vi "rszvl_core_global.vi"() -> ()   [LabVIEW 2014] (continued)
L8\r\nModifMinMaxAver: Min,Max,Aver\r\n\nRemote-control command(s):\nCALCulate<1|2>:LIMit<1>:BURSt:EVM:DATA<[:AVERage] | :MAXimum>", "Flags"={"OPC Wait"=FALSE, "Dont check status"=FALSE, "*WAI"=FALSE}, "Check Status Callback"=""}, {"Level"=3, "Descriptive Name"="WLAN Pilot Carrier EVM Limit", "Class Only"=FALSE, "Data Type"=1, "Access"=2, "Identifier"="RSZVL_ATTR_WLAN_EVM_PIL", "Range Table"="", "Command"="CALC{Window}:LIM{Limit}:BURS:EVM:PIL:{ModifMinMaxAver}", "Read Callback"="", "Write Callback"="", "Range Callback"="", "Check Callback"="", "Rngtable Callback"="", "Coerce Callback"="", "User Callback"="", "Supported Models"="", "Instrument Options"="", "Repeated Capabilities"="", "Restricted Repeated Capabilities"="", "Help"="This attribute sets the Error Vector Magnitude limit summary for the pilot carriers in dB.\n\nAvailable Repeated Capabilities:\nWindow: Win1,Win2\r\nLimit: L1,L2,L3,L4,L5,L6,L7,L8\r\nModifMinMaxAver: Min,Max,Aver\r\n\nRemote-control command(s):\nCALCulate<1|2>:LIMit<1>:BURSt:EVM:PILot<[:AVERage] | :MAXimum>", "Flags"={"OPC Wait"=FALSE, "Dont check status"=FALSE, "*WAI"=FALSE}, "Check Status Callback"=""}, {"Level"=2, "Descriptive Name"="Limit Results", "Class Only"=TRUE, "Data Type"=0, "Access"=0, "Identifier"="", "Range Table"="", "Command"="", "Read Callback"="", "Write Callback"="", "Range Callback"="", "Check Callback"="", "Rngtable Callback"="", "Coerce Callback"="", "User Callback"="", "Supported Models"="", "Instrument Options"="", "Repeated Capabilities"="", "Restricted Repeated Capabilities"="", "Help"="Attributes that return the limit results.\n\n(1) WLAN Get Fall Time Limit Result:\nThis attribute returns the fall time limit result.\n\nNote:\n(1) This attribute is valid only if standard IEEE 802.11b is selected.\n\n(2) WLAN Get Rise Time Limit Result:\nThis attribute returns the rise time limit result.\n\nNote:\n(1) This attribute is valid only if standard IEEE 802.11b is selected.\n\n(3) WLAN Get Frequency Error Limit Result:\nThis attribute returns the frequency error limit result.\n\n(4) WLAN Get Symbol Error Limit Result:\nThis attribute returns the symbol error limit result.\n\n(5) WLAN Get IQ Offset Error Limit Result:\nThis attribute returns the IQ offset error limit result.\n\n(6) WLAN Get Error Vector Magnitude Limit Result:\nThis attribute returns the Error Vector Magnitude Limit result.\n\nNote:\n(1) This attribute is available only for IEEE 802.11b standard.\n\n(7) WLAN Get Limit Check Result:\nThis attribute queries the result of the limit check of the limit line indicated in the selected\nmeasurement window. The result of the limit check responds with 0 for PASS and 1 for FAIL.\n\n\n\n(8) WLAN Get Combined EVM Limit Result:\nThis attribute returns the Error Vector Magnitude Limit result. This is a combined figure that represents the pilot, data and the free carrier.\n\n(9) WLAN Get Data Carrier EVM Limit Result:\nThis attribute returns the Error Vector Magnitude limit result summary for the data carrier in dB.\n\nValid Range:\n0 - Failed\n1 - Passed\n\n(10) WLAN Get Pilot Carrier EVM Limit Result:\nThis attribute returns the Error Vector Magnitude limit result summary for the pilot carriers in dB.\n\nValid Range:\n0 - Failed\n1 - Passed\n\n(11) WLAN Get ACP Adjacent Channel Limit:\nThis attribute returns the ACP adjacent channel limit.\n\nNote:\n(1) This attribute is available only if IEEE 802.11j is defined.\n\n(12) WLAN Get ACP Adjacent Channel Limit Result:\nThis attribute returns the ACP adjacent channel limit for IEEE 802.11j result summary (PASSED |\nFAILED) for both the lower and upper adjacent channels.\n\nNote:\n(1) This attribute is available only if IEEE 802.11j is defined.\n\n(13) WLAN Get ACP Alternate Channel Limit:\nThis attribute returns the ACP alternate channel limit.\n\nNote:\n(1) This attribute is available only if IEEE 802.11j is defined.\n\n(14) WLAN Get ACP Alternate Channel Limit Result:\nThis attribute returns the returns the ACP alternate channel limit result.\n\nNote:\n(1) This attribute is available only if IEEE 802.11j is defined.\n\n(15) WLAN Get Spectrum Max Oversteping Frequency:\nThis attribute returns the X-value at the maximum overstepping of the spectrum mask limits.\n\n(16) WLAN Get Spectrum Max Oversteping Power:\nThis attribute returns the Y-value at the maximum overstepping of the spectrum mask limits.", "Flags"={"OPC Wait"=FALSE, "Dont check status"=FALSE, "*WAI"=FALSE}, "Check Status Callback"=""}, {"Level"=3, "Descriptive Name"="WLAN Get Fall Time Limit Result", "Class Only"=FALSE, "Data Type"=0, "Access"=0, "Identifier"="RSZVL_ATTR_WLAN_TFAL_RES", "Range Table"="rszvl_rngResults", "Command"="CALC{Window}:LIM{Limit}:BURS:TFALl:{ModifMinMaxAver}:RES?", "Read Callback"="", "Write Callback"="", "Range Callback"="", "Check Callback"="", "Rngtable Callback"="", "Coerce Callback"="", "User Callback"="", "Supported Models"="", "Instrument Options"="", "Repeated Capabilities"="", "Restricted Repeated Capabilities"="", "Help"="This attribute returns the fall time limit result.\n\nNote:\n(1) This attribute is valid only if standard IEEE 802.11b is selected.\n\nAvailable Repeated Capabilities:\nWindow: Win1,Win2\r\nLimit: L1,L2,L3,L4,L5,L6,L7,L8\r\nModifMinMaxAver: Min,Max,Aver\r\n\nRemote-control command(s):\nCALCulate<1|2>:LIMit<1>:BURSt:TFALl<[:AVERage] | :MAXimum>:RESult?", "Flags"={"OPC Wait"=FALSE, "Dont check status"=FALSE, "*WAI"=FALSE}, "Check Status Callback"=""}, {"Level"=3, "Descriptive Name"="WLAN Get Rise Time Limit Result", "Class Only"=FALSE, "Data Type"=0, "Access"=0, "Identifier"="RSZVL_ATTR_WLAN_TRIS_RES", "Range Table"="rszvl_rngResults", "Command"="CALC{Window}:LIM{Limit}:BURS:TRIS:{ModifMinMaxAver}:RES?", "Read Callback"="", "Write Callback"="", "Range Callback"="", "Check Callback"="", "Rngtable Callback"="", "Coerce Callback"="", "User Callback"="", "Supported Models"="", "Instrument Options"="", "Repeated Capabilities"="", "Restricted Repeated Capabilities"="", "Help"="This attribute returns the rise time limit result.\n\nNote:\n(1) This attribute is valid only if standard IEEE 802.11b is selected.\n\nAvailable Repeated Capabilities:\nWindow: Win1,Win2\r\nLimit: L1,L2,L3,L4,L5,L6,L7,L8\r\nModifMinMaxAver: Min,Max,Aver\r\n\nRemote-control command(s):\nCALCulate<1|2>:LIMit<1>:BURSt:TRISe<[:AVERage] | :MAXimum>:RESult?", "Flags"={"OPC Wait"=FALSE, "Dont check status"=FALSE, "*WAI"=FALSE}, "Check Status Callback"=""}, {"Level"=3, "Descriptive Name"="WLAN Get Frequency Error Limit Result", "Class Only"=FALSE, "Data Type"=0, "Access"=0, "Identifier"="RSZVL_ATTR_WLAN_FERR_RES", "Range Table"="rszvl_rngResults", "Command"="CALC{Window}:LIM{Limit}:BURS:FERR:{ModifMinMaxAver}:RES?", "Read Callback"="", "Write Callback"="", "Range Callback"="", "Check Callback"="", "Rngtable Callback"="", "Coerce Callback"="", "User Callback"="", "Supported Models"="", "Instrument Options"="", "Repeated Capabilities"="", "Restricted Repeated Capabilities"="", "Help"="This attribute returns the frequency error limit result.\n\nAvailable Repeated Capabilities:\nWindow: Win1,Win2\r\nLimit: L1,L2,L3,L4,L5,L6,L7,L8\r\nModifMinMaxAver: Min,Max,Aver\r\n\nRemote-control command(s):\nCALCulate<1|2>:LIMit<1>:BURSt:FERRor<[:AVERage] | :MAXimum>:RESult?", "Flags"={"OPC Wait"=FALSE, "Dont check status"=FALSE, "*WAI"=FALSE}, "Check Status Callback"=""}, {"Level"=3, "Descriptive Name"="WLAN Get Symbol Error Limit Result", "Class Only"=FALSE, "Data Type"=0, "Access"=0, "Identifier"="RSZVL_ATTR_WLAN_SYMB_RES", "Range Table"="rszvl_rngResults", "Command"="CALC{Window}:LIM{Limit}:BURS:SYMB:{ModifMinMaxAver}:RES?", "Read Callback"="", "Write Callback"="", "Range Callback"="", "Check Callback"="", "Rngtable Callback"="", "Coerce Callback"="", "User Callback"="", "Supported Models"="", "Instrument Options"="", "Repeated Capabilities"="", "Restricted Repeated Capabilities"="", "Help"="This attribute returns the symbol error limit result.\n\nAvailable Repeated Capabilities:\nWindow: Win1,Win2\r\nLimit: L1,L2,L3,L4,L5,L6,L7,L8\r\nModifMinMaxAver: Min,Max,Aver\r\n\nRemote-control command(s):\nCALCulate<1|2>:LIMit<1>:BURSt:SYMBolerror<[:AVERage] | :MAXimum>:RESult?", "Flags"={"OPC Wait"=FALSE, "Dont check status"=FALSE, "*WAI"=FALSE}, "Check Status Callback"=""}, {"Level"=3, "Descriptive Name"="WLAN Get IQ Offset Error Limit Result", "Class Only"=FALSE, "Data Type"=0, "Access"=0, "Identifier"="RSZVL_ATTR_WLAN_IQOF_RES", "Range Table"="rszvl_rngResults", "Command"="CALC{Window}:LIM{Limit}:BURS:IQOF:{ModifMinMaxAver}:RES?", "Read Callback"="", "Write Callback"="", "Range Callback"="", "Check Callback"="", "Rngtable Callback"="", "Coerce Callback"="", "User Callback"="", "Supported Models"="", "Instrument Options"="", "Repeated Capabilities"="", "Restricted Repeated Capabilities"="", "Help"="This attribute returns the IQ offset error limit result.\n\nAvailable Repeated Capabilities:\nWindow: Win1,Win2\r\nLimit: L1,L2,L3,L4,L5,L6,L7,L8\r\nModifMinMaxAver: Min,Max,Aver\r\n\nRemote-control command(s):\nCALCulate<1|2>:LIMit<1>:BURSt:IQOFfset<[:AVERage] | :MAXimum>:RESult?", "Flags"={"OPC Wait"=FALSE, "Dont check status"=FALSE, "*WAI"=FALSE}, "Check Status Callback"=""}, {"Level"=3, "Descriptive Name"="WLAN Get Error Vector Magnitude Limit Result", "Class Only"=FALSE, "Data Type"=0, "Access"=0, "Identifier"="RSZVL_ATTR_WLAN_EVM_RES", "Range Table"="rszvl_rngResults", "Command"="CALC{Window}:LIM{Limit}:BURS:EVM:{ModifMinMaxAver}:RES?", "Read Callback"="", "Write Callback"="", "Range Callback"="", "Check Callback"="", "Rngtable Callback"="", "Coerce Callback"="", "User Callback"="", "Supported Models"="", "Instrument Options"="", "Repeated Capabilities"="", "Restricted Repeated Capabilities"="", "Help"="This attribute returns the Error Vector Magnitude Limit result.\n\nNote:\n(1) This attribute is available only for IEEE 802.11b standard.\n\nAvailable Repeated Capabilities:\nWindow: Win1,Win2\r\nLimit: L1,L2,L3,L4,L5,L6,L7,L8\r\nModifMinMaxAver: Min,Max,Aver\r\n\nRemote-control command(s):\nCALCulate<1|2>:LIMit<1>:BURSt:EVM<[:AVERage] | :MAXimum>:RESult?", "Flags"={"OPC Wait"=FALSE, "Dont check status"=FALSE, "*WAI"=FALSE}, "Check Status Callback"=""}, {"Level"=3, "Descriptive Name"="WLAN Get Limit Check Result", "Class Only"=FALSE, "Data Type"=0, "Access"=0, "Identifier"="RSZVL_ATTR_WLAN_LIM_FAIL_RES", "Range Table"="", "Command"="CALC{Window}:LIM{Limit}:FAIL?", "Read Callback"="", "Write Callback"="", "Range Callback"="", "Check Callback"="", "Rngtable Callback"="", "Coerce Callback"="", "User Callback"="", "Supported Models"="", "Instrument Options"="", "Repeated Capabilities"="", "Restricted Repeated Capabilities"="", "Help"="This attribute queries the result of the limit check of the limit line indicated in the selected\nmeasurement window. The result of the limit check responds with 0 for PASS and 1 for FAIL.\n\nAvailable Repeated Capabilities:\nWindow: Win1,Win2\r\nLimit: L1,L2,L3,L4,L5,L6,L7,L8\r\n\nRemote-control command(s):\nCALCulate<1|2>:LIMit<1>:FAIL?", "Flags"={"OPC Wait"=FALSE, "Dont check status"=FALSE, "*WAI"=FALSE}, "Check Status Callback"=""}, {"Level"=3, "Descriptive Name"="WLAN Get Combined EVM Limit Result", "Class Only"=FALSE, "Data Type"=0, "Access"=0, "Identifier"="RSZVL_ATTR_WLAN_EVM_ALL_RES", "Range Table"="rszvl_rngResults", "Command"="CALC{Window}:LIM{Limit}:BURS:EVM:ALL:{ModifMinMaxAver}:RES?", "Read Callback"="", "Write Callback"="", "Range Callback"="", "Check Callback"="", "Rngtable Callback"="", "Coerce Callback"="", "User Callback"="", "Supported Models"="", "Instrument Options"="", "Repeated Capabilities"="", "Restricted Repeated Capabilities"="", "Help"="This attribute returns the Error Vector Magnitude Limit result. This is a combined figure that represents the pilot, data and the free carrier.\n\nAvailable Repeated Capabilities:\nWindow: Win1,Win2\r\nLimit: L1,L2,L3,L4,L5,L6,L7,L8\r\nModifMinMaxAver: Min,Max,Aver\r\n\nRemote-control command(s):\nCALCulate<1|2>:LIMit<1>:BURSt:EVM:ALL<[:AVERage] | :MAXimum>:RESult?", "Flags"={"OPC Wait"=FALSE, "Dont check status"=FALSE, "*WAI"=FALSE}, "Check Status Callback"=""}, {"Level"=3, "Descriptive Name"="WLAN Get Data Carrier EVM Limit Result", "Class Only"=FALSE, "Data Type"=0, "Access"=0, "Identifier"="RSZVL_ATTR_WLAN_EVM_DATA_RES", "Range Table"="rszvl_rngResults", "Command"="CALC{Window}:LIM{Limit}:BURS:EVM:DATA:{ModifMinMaxAver}:RES?", "Read Callback"="", "Write Callback"="", "Range Callback"="", "Check Callback"="", "Rngtable Callback"="", "Coerce Callback"="", "User Callback"="", "Supported Models"="", "Instrument Options"="", "Repeated Capabilities"="", "Restricted Repeated Capabilities"="", "Help"="This attribute returns the Error Vector Magnitude limit result summary for the data carrier in dB.\n\nValid Range:\n0 - Failed\n1 - Passed\n\nAvailable Repeated Capabilities:\nWindow: Win1,Win2\r\nLimit: L1,L2,L3,L4,L5,L6,L7,L8\r\nModifMinMaxAver: Min,Max,Aver\r\n\nRemote-control command(s):\nCALCulate<1|2>:LIMit<1>:BURSt:EVM:DATA<[:AVERage] | :MAXimum>:RESult?", "Flags"={"OPC Wait"=FALSE, "Dont check status"=FALSE, "*WAI"=FALSE}, "Check Status Callback"=""}, {"Level"=3, "Descriptive Name"="WLAN Get Pilot Carrier EVM Limit Result", "Class Only"=FALSE, "Data Type"=0, "Access"=0, "Identifier"="RSZVL_ATTR_WLAN_EVM_PIL_RES", "Range Table"="rszvl_rngResults", "Command"="CALC{Window}:LIM{Limit}:BURS:EVM:PIL:{ModifMinMaxAver}:RES?", "Read Callback"="", "Write Callback"="", "Range Callback"="", "Check Callback"="", "Rngtable Callback"="", "Coerce Callback"="", "User Callback"="", "Supported Models"="", "Instrument Options"="", "Repeated Capabilities"="", "Restricted Repeated Capabilities"="", "Help"="This attribute returns the Error Vector Magnitude limit result summary for the pilot carriers in dB.\n\nValid Range:\n0 - Failed\n1 - Passed\n\nAvailable Repeated Capabilities:\nWindow: Win1,Win2\r\nLimit: L1,L2,L3,L4,L5,L6,L7,L8\r\nModifMinMaxAver: Min,Max,Aver\r\n\nRemote-control command(s):\nCALCulate<1|2>:LIMit<1>:BURSt:EVM:PILot<[:AVERage] | :MAXimum>:RESult?", "Flags"={"OPC Wait"=FALSE, "Dont check status"=FALSE, "*WAI"=FALSE}, "Check Status Callback"=""}, {"Level"=3, "Descriptive Name"="WLAN Get ACP Adjacent Channel Limit", "Class Only"=FALSE, "Data Type"=1, "Access"=0, "Identifier"="RSZVL_ATTR_WLAN_ACP_ADJ", "Range Table"="", "Command"="CALC{Window}:LIM{Limit}:ACP:ACH?", "Read Callback"="", "Write Callback"="", "Range Callback"="", "Check Callback"="", "Rngtable Callback"="", "Coerce Callback"="", "User Callback"="", "Supported Models"="", "Instrument Options"="", "Repeated Capabilities"="", "Restricted Repeated Capabilities"="", "Help"="This attribute returns the ACP adjacent channel limit.\n\nNote:\n(1) This attribute is available only if IEEE 802.11j is defined.\n\nAvailable Repeated Capabilities:\nWindow: Win1,Win2\r\nLimit: L1,L2,L3,L4,L5,L6,L7,L8\r\n\nRemote-control command(s):\nCALCulate<1|2>:LIMit<1>:ACPower:ACHannel?", "Flags"={"OPC Wait"=FALSE, "Dont check status"=FALSE, "*WAI"=FALSE}, "Check Status Callback"=""}, {"Level"=3, "Descriptive Name"="WLAN Get ACP Adjacent Channel Limit Result", "Class Only"=FALSE, "Data Type"=0, "Access"=0, "Identifier"="RSZVL_ATTR_WLAN_ACP_ADJ_RES", "Range Table"="rszvl_rngResults", "Command"="CALC{Window}:LIM{Limit}:ACP:ACH:RES?", "Read Callback"="", "Write Callback"="", "Range Callback"="", "Check Callback"="", "Rngtable Callback"="", "Coerce Callback"="", "User Callback"="", "Supported Models"="", "Instrument Options"="", "Repeated Capabilities"="", "Restricted Repeated Capabilities"="", "Help"="This attribute returns the ACP adjacent channel limit for IEEE 802.11j result summary (PASSED |\nFAILED) for both the lower and upper adjacent channels.\n\nNote:\n(1) This attribute is available only if IEEE 802.11j is defined.\n\nAvailable Repeated Capabilities:\nWindow: Win1,Win2\r\nLimit: L1,L2,L3,L4,L5,L6,L7,L8\r\n\nRemote-control command(s):\nCALCulate<1|2>:LIMit<1>:ACPower:ACHannel:RESult?", "Flags"={"OPC Wait"=FALSE, "Dont check status"=FALSE, "*WAI"=FALSE}, "Check Status Callback"=""}, {"Level"=3, "Descriptive Name"="WLAN Get ACP Alternate Channel Limit", "Class Only"=FALSE, "Data Type"=1, "Access"=0, "Identifier"="RSZVL_ATTR_WLAN_ACP_ALT", "Range Table"="", "Command"="CALC{Window}:LIM{Limit}:ACP:ALT?", "Read Callback"="", "Write Callback"="", "Range Callback"="", "Check Callback"="", "Rngtable Callback"="", "Coerce Callback"="", "User Callback"="", "Supported Models"="", "Instrument Options"="", "Repeated Capabilities"="", "Restricted Repeated Capabilities"="", "Help"="This attribute returns the ACP alternate channel limit.\n\nNote:\n(1) This attribute is available only if IEEE 802.11j is defined.\n\nAvailable Repeated Capabilities:\nWindow: Win1,Win2\r\nLimit: L1,L2,L3,L4,L5,L6,L7,L8\r\n\nRemote-control command(s):\nCALCulate<1|2>:LIMit<1>:ACPower:ALTernate?", "Flags"={"OPC Wait"=FALSE, "Dont check status"=FALSE, "*WAI"=FALSE}, "Check Status Callback"=""}, {"Level"=3, "Descriptive Name"="WLAN Get ACP Alternate Channel Limit Result", "Class Only"=FALSE, "Data Type"=0, "Access"=0, "Identifier"="RSZVL_ATTR_WLAN_ACP_ALT_RES", "Range Table"="rszvl_rngResults", "Command"="CALC{Window}:LIM{Limit}:ACP:ALT:RES?", "Read Callback"="", "Write Callback"="", "Range Callback"="", "Check Callback"="", "Rngtable Callback"="", "Coerce Callback"="", "User Callback"="", "Supported Models"="", "Instrument Options"="", "Repeated Capabilities"="", "Restricted Repeated Capabilities"="", "Help"="This attribute returns the returns the ACP alternate channel limit result.\n\nNote:\n(1) This attribute is available only if IEEE 802.11j is defined.\n\nAvailable Repeated Capabilities:\nWindow: Win1,Win2\r\nLimit: L1,L2,L3,L4,L5,L6,L7,L8\r\n\nRemote-control command(s):\nCALCulate<1|2>:LIMit<1>:ACPower:ALTernate:RESult?", "Flags"={"OPC Wait"=FALSE, "Dont check status"=FALSE, "*WAI"=FALSE}, "Check Status Callback"=""}, {"Level"=3, "Descriptive Name"="WLAN Get Spectrum Max Oversteping Frequency", "Class Only"=FALSE, "Data Type"=1, "Access"=0, "Identifier"="RSZVL_ATTR_WLAN_SPEC_MASK_X", "Range Table"="", "Command"="CALC{Window}:LIM{Limit}:SPEC:MASK:CHEC:X?", "Read Callback"="", "Write Callback"="", "Range Callback"="", "Check Callback"="", "Rngtable Callback"="", "Coerce Callback"="", "User Callback"="", "Supported Models"="", "Instrument Options"="", "Repeated Capabilities"="", "Restricted Repeated Capabilities"="", "Help"="This attribute returns the X-value at the maximum overstepping of the spectrum mask limits.\n\nAvailable Repeated Capabilities:\nWindow: Win1,Win2\r\nLimit: L1,L2,L3,L4,L5,L6,L7,L8\r\n\nRemote-control command(s):\nCALCulate<1|2>:LIMit<1>:SPECtrum:MASK:CHECk:X?", "Flags"={"OPC Wait"=FALSE, "Dont check status"=FALSE, "*WAI"=FALSE}, "Check Status Callback"=""}, {"Level"=3, "Descriptive Name"="WLAN Get Spectrum Max Oversteping Power", "Class Only"=FALSE, "Data Type"=1, "Access"=0, "Identifier"="RSZVL_ATTR_WLAN_SPEC_MASK_Y", "Range Table"="", "Command"="CALC{Window}:LIM{Limit}:SPEC:MASK:CHEC:Y?", "Read Callback"="", "Write Callback"="", "Range Callback"="", "Check Callback"="", "Rngtable Callback"="", "Coerce Callback"="", "User Callback"="", "Supported Models"="", "Instrument Options"="", "Repeated Capabilities"="", "Restricted Repeated Capabilities"="", "Help"="This attribute returns the Y-value at the maximum overstepping of the spectrum mask limits.\n\nAvailable Repeated Capabilities:\nWindow: Win1,Win2\r\nLimit: L1,L2,L3,L4,L5,L6,L7,L8\r\n\nRemote-control command(s):\nCALCulate<1|2>:LIMit<1>:SPECtrum:MASK:CHECk:Y?", "Flags"={"OPC Wait"=FALSE, "Dont check status"=FALSE, "*WAI"=FALSE}, "Check Status Callback"=""}, {"Level"=2, "Descriptive Name"="Marker Settings", "Class Only"=TRUE, "Data Type"=0, "Access"=0, "Identifier"="", "Range Table"="", "Command"="", "Read Callback"="", "Write Callback"="", "Range Callback"="", "Check Callback"="", "Rngtable Callback"="", "Coerce Callback"="", "User Callback"="", "Supported Models"="", "Instrument Options"="", "Repeated Capabilities"="", "Restricted Repeated Capabilities"="", "Help"="Attributes that configure the marker settings.\n\n(1) WLAN Marker Symbol:\nThis attribute positions the selected marker to the indicated quadrature (constellation Vs symbol), magnitude of I or Q (constellation Vs carrier), EVM (EVM Vs carrier) or abs (spectrum flatness) in the selected measurement window.\n\nNote:\n(1) This attribute is query only for the following result displays:\n- Auto level\n- Constellation Vs Symbol\n- Constellation Vs Carrier\n- EVM Vs Symbol\n- PVT Full\n- PVT Rising / Falling\n- Magnitude Capture Buffer\n- Spectrum Mask\n- Spectrum ACP/ACPR\n- Spectrum FFT\n- CCDF\n\n(2) WLAN Marker Carrier:\nThis attribute positions the selected marker to the indicated quadrature (constellation Vs symbol), magnitude of I or Q (constellation Vs carrier), EVM (EVM Vs carrier) or abs (spectrum flatness) in the selected measurement window.\n\nNote:\n(1) This attribute is query only for the following result displays:\n- Auto level\n- Constellation Vs Symbol\n- Constellation Vs Carrier\n- EVM Vs Symbol\n- PVT Full\n- PVT Rising / Falling\n- Magnitude Capture Buffer\n- Spectrum Mask\n- Spectrum ACP/ACPR\n- Spectrum FFT\n- CCDF\n\n(3) WLAN Marker Position Y:\nThis attribute positions the selected marker to the indicated quadrature (constellation Vs symbol), magnitude of I or Q (constellation Vs carrier), EVM (EVM Vs carrier) or abs (spectrum flatness) in the selected measurement window.\n\nNote:\n(1) This attribute is query only for the following result displays:\n- Auto level\n- Constellation Vs Symbol\n- Constellation Vs Carrier\n- EVM Vs Symbol\n- PVT Full\n- PVT Rising / Falling\n- Magnitude Capture Buffer\n- Spectrum Mask\n- Spectrum ACP/ACPR\n- Spectrum FFT\n- CCDF", "Flags"={"OPC Wait"=FALSE, "Dont check status"=FALSE, "*WAI"=FALSE}, "Check Status Callback"=""}, {"Level"=3, "Descriptive Name"="WLAN Marker State", "Class Only"=FALSE, "Data Type"=3, "Access"=2, "Identifier"="RSZVL_ATTR_WLAN_MARKER_ENABLED", "Range Table"="", "Command"="CALC{Window}:MARK{Marker}:STAT", "Read Callback"="", "Write Callback"="", "Range Callback"="", "Check Callback"="", "Rngtable Callback"="", "Coerce Callback"="", "User Callback"="", "Supported Models"="", "Instrument Options"="", "Repeated Capabilities"="", "Restricted Repeated Capabilities"="", "Help"="This attribute switches on or off the currently selected marker. If no indication is made, marker 1 is selected automatically. If marker 2, 3 or 4 is selected and used as a delta marker, it is switched to marker mode.\n\nAvailable Repeated Capabilities:\nWindow: Win1,Win2\r\nMarker: M1,M2,M3,M4\r\n\nRemote-control command(s):\nCALCulate<1|2>:MARKer<1 to 4>[:STATe]", "Flags"={"OPC Wait"=FALSE, "Dont check status"=FALSE, "*WAI"=FALSE}, "Check Status Callback"=""}, {"Level"=3, "Descriptive Name"="WLAN All Markers Off", "Class Only"=FALSE, "Data Type"=4, "Access"=1, "Identifier"="RSZVL_ATTR_WLAN_MARKERS_AOFF", "Range Table"="", "Command"="CALC{Window}:MARK:AOFF", "Read Callback"="", "Write Callback"="", "Range Callback"="", "Check Callback"="", "Rngtable Callback"="", "Coerce Callback"="", "User Callback"="", "Supported Models"="", "Instrument Options"="", "Repeated Capabilities"="", "Restricted Repeated Capabilities"="", "Help"="This attribute switches off all active markers.\n\nAvailable Repeated Capabilities:\nWindow: Win1,Win2\r\n\nRemote-control command(s):\nCALCulate<1|2>:MARKer<1 to 4>:AOFF", "Flags"={"OPC Wait"=FALSE, "Dont check status"=FALSE, "*WAI"=FALSE}, "Check Status Callback"=""}, {"Level"=3, "Descriptive Name"="WLAN Assign Marker to Trace", "Class Only"=FALSE, "Data Type"=0, "Access"=2, "Identifier"="RSZVL_ATTR_WLAN_MARKER_TRACE", "Range Table"="rszvl_rngTrace", "Command"="CALC{Window}:MARK{Marker}:TRAC", "Read Callback"="", "Write Callback"="", "Range Callback"="", "Check Callback"="", "Rngtable Callback"="", "Coerce Callback"="", "User Callback"="", "Supported Models"="", "Instrument Options"="", "Repeated Capabilities"="", "Restricted Repeated Capabilities"="", "Help"="This attribute assigns the selected marker to the indicated measurement curve. The corresponding trace must be active, i.e. its status must be different from BLANK.\n\nAvailable Repeated Capabilities:\nWindow: Win1,Win2\r\nMarker: M1,M2,M3,M4\r\n\nRemote-control command(s):\nCALCulate<1|2>:MARKer<1 to 4>:TRACe", "Flags"={"OPC Wait"=FALSE, "Dont check status"=FALSE, "*WAI"=FALSE}, "Check Status Callback"=""}, {"Level"=3, "Descriptive Name"="WLAN Marker Symbol", "Class Only"=FALSE, "Data Type"=0, "Access"=2, "Identifier"="RSZVL_ATTR_WLAN_MARK_SYMB", "Range Table"="", "Command"="CALC{Window}:MARK{Marker}:SYMB", "Read Callback"="", "Write Callback"="", "Range Callback"="", "Check Callback"="", "Rngtable Callback"="", "Coerce Callback"="", "User Callback"="", "Supported Models"="", "Instrument Options"="", "Repeated Capabilities"="", "Restricted Repeated Capabilities"="", "Help"="This attribute positions the selected marker to the indicated quadrature (constellation Vs symbol), magnitude of I or Q (constellation Vs carrier), EVM (EVM Vs carrier) or abs (spectrum flatness) in the selected measurement window.\n\nNote:\n(1) This attribute is query only for the following result displays:\n- Auto level\n- Constellation Vs Symbol\n- Constellation Vs Carrier\n- EVM Vs Symbol\n- PVT Full\n- PVT Rising / Falling\n- Magnitude Capture Buffer\n- Spectrum Mask\n- Spectrum ACP/ACPR\n- Spectrum FFT\n- CCDF\n\nAvailable Repeated Capabilities:\nWindow: Win1,Win2\r\nMarker: M1,M2,M3,M4\r\n\nRemote-control command(s):\nCALCulate<1|2>:MARKer<1>:SYMBol", "Flags"={"OPC Wait"=FALSE, "Dont check status"=FALSE, "*WAI"=FALSE}, "Check Status Callback"=""}, {"Level"=3, "Descriptive Name"="WLAN Marker Carrier", "Class Only"=FALSE, "Data Type"=0, "Access"=2, "Identifier"="RSZVL_ATTR_WLAN_MARK_CARR", "Range Table"="", "Command"="CALC{Window}:MARK{Marker}:CARR", "Read Callback"="", "Write Callback"="", "Range Callback"="", "Check Callback"="", "Rngtable Callback"="", "Coerce Callback"="", "User Callback"="", "Supported Models"="", "Instrument Options"="", "Repeated Capabilities"="", "Restricted Repeated Capabilities"="", "Help"="This attribute positions the selected marker to the indicated quadrature (constellation Vs symbol), magnitude of I or Q (constellation Vs carrier), EVM (EVM Vs carrier) or abs (spectrum flatness) in the selected measurement window.\n\nNote:\n(1) This attribute is query only for the following result displays:\n- Auto level\n- Constellation Vs Symbol\n- Constellation Vs Carrier\n- EVM Vs Symbol\n- PVT Full\n- PVT Rising / Falling\n- Magnitude Capture Buffer\n- Spectrum Mask\n- Spectrum ACP/ACPR\n- Spectrum FFT\n- CCDF\n\nAvailable Repeated Capabilities:\nWindow: Win1,Win2\r\nMarker: M1,M2,M3,M4\r\n\nRemote-control command(s):\nCALCulate<1|2>:MARKer<1>:CARRier", "Flags"={"OPC Wait"=FALSE, "Dont check status"=FALSE, "*WAI"=FALSE}, "Check Status Callback"=""}, {"Level"=3, "Descriptive Name"="WLAN Marker Position Y", "Class Only"=FALSE, "Data Type"=1, "Access"=2, "Identifier"="RSZVL_ATTR_WLAN_MARK_Y", "Range Table"="", "Command"="CALC{Window}:MARK{Marker}:Y", "Read Callback"="", "Write Callback"="", "Range Callback"="", "Check Callback"="", "Rngtable Callback"="", "Coerce Callback"="", "User Callback"="", "Supported Models"="", "Instrument Options"="", "Repeated Capabilities"="", "Restricted Repeated Capabilities"="", "Help"="This attribute positions the selected marker to the indicated quadrature (constellation Vs symbol), magnitude of I or Q (constellation Vs carrier), EVM (EVM Vs carrier) or abs (spectrum flatness) in the selected measurement window.\n\nNote:\n(1) This attribute is query only for the following result displays:\n- Auto level\n- Constellation Vs Symbol\n- Constellation Vs Carrier\n- EVM Vs Symbol\n- PVT Full\n- PVT Rising / Falling\n- Magnitude Capture Buffer\n- Spectrum Mask\n- Spectrum ACP/ACPR\n- Spectrum FFT\n- CCDF\n\nAvailable Repeated Capabilities:\nWindow: Win1,Win2\r\nMarker: M1,M2,M3,M4\r\n\nRemote-control command(s):\nCALCulate<1|2>:MARKer<1>:Y", "Flags"={"OPC Wait"=FALSE, "Dont check status"=FALSE, "*WAI"=FALSE}, "Check Status Callback"=""}, {"Level"=3, "Descriptive Name"="WLAN Marker Position X", "Class Only"=FALSE, "Data Type"=1, "Access"=2, "Identifier"="RSZVL_ATTR_WLAN_MARKER_POSITION", "Range Table"="", "Command"="CALC{Window}:MARK{Marker}:X", "Read Callback"="", "Write Callback"="", "Range Callback"="", "Check Callback"="", "Rngtable Callback"="", "Coerce Callback"="", "User Callback"="", "Supported Models"="", "Instrument Options"="", "Repeated Capabilities"="", "Restricted Repeated Capabilities"="", "Help"="This attribute positions the selected marker to the indicated frequency (span > 0), time (span = 0) or level (APD measurement or CCDF measurement ON). If marker 2, 3 or 4 is selected and used as delta marker, it is switched to marker mode.\n\nAvailable Repeated Capabilities:\nWindow: Win1,Win2\r\nMarker: M1,M2,M3,M4\r\n\nRemote-control command(s):\nCALCulate<1|2>:MARKer<1 to 4>:X", "Flags"={"OPC Wait"=FALSE, "Dont check status"=FALSE, "*WAI"=FALSE}, "Check Status Callback"=""}, {"Level"=3, "Descriptive Name"="WLAN Marker Zoom", "Class Only"=FALSE, "Data Type"=1, "Access"=2, "Identifier"="RSZVL_ATTR_WLAN_MARKER_ZOOM", "Range Table"="", "Command"="CALC{Window}:MARK{Marker}:FUNC:ZOOM", "Read Callback"="", "Write Callback"="", "Range Callback"="", "Check Callback"="", "Rngtable Callback"="", "Coerce Callback"="", "User Callback"="", "Supported Models"="", "Instrument Options"="", "Repeated Capabilities"="", "Restricted Repeated Capabilities"="", "Help"="This attribute defines the range to be zoomed around marker 1. Marker 1 is activated first, if necessary.\nThe subsequent frequency sweep is stopped at the marker position and the frequency of the signal is counted. This frequency becomes the new center frequency, and the zoomed span is set. In order to recognize the end of the operation the synchronization to the sweep end should be activated. This is only possible in single sweep mode.\n\nAvailable Repeated Capabilities:\nWindow: Win1,Win2\r\nMarker: M1,M2,M3,M4\r\n\nRemote-control command(s):\nCALCulate<1|2>:MARKer<1 to 4>:FUNCtion:ZOOM", "Flags"={"OPC Wait"=FALSE, "Dont check status"=FALSE, "*WAI"=FALSE}, "Check Status Callback"=""}, {"Level"=3, "Descriptive Name"="WLAN Marker Search Peak Maximum", "Class Only"=FALSE, "Data Type"=4, "Access"=1, "Identifier"="RSZVL_ATTR_WLAN_MARKER_SEARCH_MAX", "Range Table"="", "Command"="CALC{Window}:MARK{Marker}:MAX", "Read Callback"="", "Write Callback"="", "Range Callback"="", "Check Callback"="", "Rngtable Callback"="", "Coerce Callback"="", "User Callback"="", "Supported Models"="", "Instrument Options"="", "Repeated Capabilities"="", "Restricted Repeated Capabilities"="", "Help"="This attribute positions the marker to the current maximum value of the corresponding trace. The corresponding marker is activated first or switched to the marker mode.\nNote: If no maximum value is found on the trace (level spacing to adjacent values < peak excursion), an execution error (error eode: -200) is produced.\n\nAvailable Repeated Capabilities:\nWindow: Win1,Win2\r\nMarker: M1,M2,M3,M4\r\n\nRemote-control command(s):\nCALCulate<1|2>:MARKer<1 to 4>:MAXimum[:PEAK]", "Flags"={"OPC Wait"=FALSE, "Dont check status"=FALSE, "*WAI"=FALSE}, "Check Status Callback"=""}, {"Level"=3, "Descriptive Name"="WLAN Marker Search Peak Minimum", "Class Only"=FALSE, "Data Type"=4, "Access"=1, "Identifier"="RSZVL_ATTR_WLAN_MARKER_SEARCH_MIN", "Range Table"="", "Command"="CALC{Window}:MARK{Marker}:MIN", "Read Callback"="", "Write Callback"="", "Range Callback"="", "Check Callback"="", "Rngtable Callback"="", "Coerce Callback"="", "User Callback"="", "Supported Models"="", "Instrument Options"="", "Repeated Capabilities"="", "Restricted Repeated Capabilities"="", "Help"="This attribute positions the marker to the current minimum value of the corresponding trace. The corresponding marker is activated first or switched to marker mode, if necessary.\n\nNote: If no minimum value is found on the trace (level spacing to adjacent values < peak excursion), an execution error (error code: -200) is produced.\n\nAvailable Repeated Capabilities:\nWindow: Win1,Win2\r\nMarker: M1,M2,M3,M4\r\n\nRemote-control command(s):\nCALCulate<1|2>:MARKer<1 to 4>:MINimum[:PEAK]", "Flags"={"OPC Wait"=FALSE, "Dont check status"=FALSE, "*WAI"=FALSE}, "Check Status Callback"=""}, {"Level"=2, "Descriptive Name"="Results", "Class Only"=TRUE, "Data Type"=0, "Access"=0, "Identifier"="", "Range Table"="", "Command"="", "Read Callback"="", "Write Callback"="", "Range Callback"="", "Check Callback"="", "Rngtable Callback"="", "Coerce Callback"="", "User Callback"="", "Supported Models"="", "Instrument Options"="", "Repeated Capabilities"="", "Restricted Repeated Capabilities"="", "Help"="Attributes that returns measurement values.\n\n(1) WLAN Fetch Burst Count:\nThis attribute returns the number of analyzed bursts\n\nFW Version 3.70\n\n(2) WLAN Fetch Preamble Power:\nThis attribute returns the measured power in the burst preamble.\n\n(3) WLAN Fetch Payload Power:\nThis attribute returns the measured power in the payload of the burst.\n\n(4) WLAN Fetch RMS Power:\nThis attribute returns the RMS burst power in dBm measured during the measurement.\n\n(5) WLAN Fetch Peak Power:\nThis attribute returns the peak power in dBm measured during the measurement time.\n\n(6) WLAN Fetch Crest Factor:\nThis attribute returns the determined CREST factor (= ratio of peak power to average power) in dB.\n\n(7) WLAN Fetch Rise Time:\nThis attribute returns the burst rise time in seconds.\n\nNote:\n(1) This attribute is valid only if standard IEEE 802.11b is selected.\n\n(8) WLAN Fetch Fall Time:\nThis attribute returns the burst fall time in seconds.\n\nNote :\n(1) This attribute is available only for IEEE 802.11b standard.\n\n(9) WLAN Fetch Frequency Error:\nThis attribute returns the measured frequency error in Hz.\n\n(10) WLAN Fetch Symbol Error:\nThis attribute returns the number of symbols  that were outside the permissible demodulation\nrange within a burst.\n\n(11) WLAN Fetch IQ Offset Error:\nThis attribute returns the measured IQ offset errors in dB.\n\n(12) WLAN Fetch IQ Imbalance Error:\nThis attribute returns the measured IQ imbalance errors in dB.\n\n(13) WLAN Fetch Quadrature Error:\nThis attribute returns the accuracy in terms of the phase error of symbols within a burst.\nIt returns the angle error recorded for a symbol during the measurement.\n\n(14) WLAN Fetch EVM:\nThis attribute returns the error vector magnitude measurement results summary in dB for the IEEE 802.11b standard. This result is the value before filtering.\n\nNote :\n(1) This attribute is available only for IEEE 802.11b standard.\n\n(15) WLAN Fetch Filtered EVM:\nThis attribute returns the error vector magnitude measurement results summary in dB for the IEEE 802.11b standard. This result is the value after filtering.\n\nNote :\n(1) This attribute is available only for IEEE 802.11b standard.\n\n(16) WLAN Fetch EVM All Carriers:\nThis attribute returns the error vector magnitude measurement results summary in dB. This is a combined figure that represents the pilot, data and the free carrier.\n\n(17) WLAN Fetch EVM Data Carriers:\nThis attribute returns the error vector magnitude measurement results summary for the data carrier\nin dB.\n\n(18) WLAN Fetch EVM Pilot Carriers:\nThis attribute returns the error vector magnitude measurement results summary for the EVM pilot\ncarrier in dB.\n\n(19) WLAN Fetch Symbol Count:\nThis attribute returns the number of symbols for each analyzed burst\n\nFW 3.70", "Flags"={"OPC Wait"=FALSE, "Dont check status"=FALSE, "*WAI"=FALSE}, "Check Status Callback"=""}, {"Level"=3, "Descriptive Name"="WLAN Fetch Burst Count", "Class Only"=FALSE, "Data Type"=0, "Access"=0, "Identifier"="RSZVL_ATTR_WLAN_FETC_BURS_COUNT", "Range Table"="", "Command"="FETC:BURS:COUNt?", "Read Callback"="", "Write Callback"="", "Range Callback"="", "Check Callback"="", "Rngtable Callback"="", "Coerce Callback"="", "User Callback"="", "Supported Models"="", "Instrument Options"="", "Repeated Capabilities"="", "Restricted Repeated Capabilities"="", "Help"="This attribute returns the number of analyzed bursts\n\nFW Version 3.70\n\nAvailable Repeated Capabilities:\nNone\n\nRemote-control command(s):\nFETCh:BURSt:COUNt?", "Flags"={"OPC Wait"=FALSE, "Dont check status"=FALSE, "*WAI"=FALSE}, "Check Status Callback"=""}, {"Level"=3, "Descriptive Name"="WLAN Fetch Preamble Power", "Class Only"=FALSE, "Data Type"=1, "Access"=0, "Identifier"="RSZVL_ATTR_WLAN_FETC_PRE", "Range Table"="", "Command"="FETC:BURS:PRE?", "Read Callback"="", "Write Callback"="", "Range Callback"="", "Check Callback"="", "Rngtable Callback"="", "Coerce Callback"="", "User Callback"="", "Supported Models"="", "Instrument Options"="", "Repeated Capabilities"="", "Restricted Repeated Capabilities"="", "Help"="This attribute returns the measured power in the burst preamble.\n\nAvailable Repeated Capabilities:\nNone\n\nRemote-control command(s):\nFETCh:BURSt:PREamble?", "Flags"={"OPC Wait"=FALSE, "Dont check status"=FALSE, "*WAI"=FALSE}, "Check Status Callback"=""}, {"Level"=3, "Descriptive Name"="WLAN Fetch Payload Power", "Class Only"=FALSE, "Data Type"=1, "Access"=0, "Identifier"="RSZVL_ATTR_WLAN_FETC_PAYL", "Range Table"="", "Command"="FETC:BURS:PAYL?", "Read Callback"="", "Write Callback"="", "Range Callback"="", "Check Callback"="", "Rngtable Callback"="", "Coerce Callback"="", "User Callback"="", "Supported Models"="", "Instrument Options"="", "Repeated Capabilities"="", "Restricted Repeated Capabilities"="", "Help"="This attribute returns the measured power in the payload of the burst.\n\nAvailable Repeated Capabilities:\nNone\n\nRemote-control command(s):\nFETCh:BURSt:PAYLoad?", "Flags"={"OPC Wait"=FALSE, "Dont check status"=FALSE, "*WAI"=FALSE}, "Check Status Callback"=""}, {"Level"=3, "Descriptive Name"="WLAN Fetch RMS Power", "Class Only"=FALSE, "Data Type"=1, "Access"=0, "Identifier"="RSZVL_ATTR_WLAN_FETC_RMS", "Range Table"="", "Command"="FETC:BURS:RMS:{ModifMinMaxAver}?", "Read Callback"="", "Write Callback"="", "Range Callback"="", "Check Callback"="", "Rngtable Callback"="", "Coerce Callback"="", "User Callback"="", "Supported Models"="", "Instrument Options"="", "Repeated Capabilities"="", "Restricted Repeated Capabilities"="", "Help"="This attribute returns the RMS burst power in dBm measured during the measurement.\n\nAvailable Repeated Capabilities:\nModifMinMaxAver: Min,Max,Aver\r\n\nRemote-control command(s):\nFETCh:BURSt:RMS:<AVERage | MAXimum | MIMimum>?", "Flags"={"OPC Wait"=FALSE, "Dont check status"=FALSE, "*WAI"=FALSE}, "Check Status Callback"=""}, {"Level"=3, "Descriptive Name"="WLAN Fetch Peak Power", "Class Only"=FALSE, "Data Type"=1, "Access"=0, "Identifier"="RSZVL_ATTR_WLAN_FETC_PEAK", "Range Table"="", "Command"="FETC:BURS:PEAK?", "Read Callback"="", "Write Callback"="", "Range Callback"="", "Check Callback"="", "Rngtable Callback"="", "Coerce Callback"="", "User Callback"="", "Supported Models"="", "Instrument Options"="", "Repeated Capabilities"="", "Restricted Repeated Capabilities"="", "Help"="This attribute returns the peak power in dBm measured during the measurement time.\n\nAvailable Repeated Capabilities:\nNone\n\nRemote-control command(s):\nFETCh:BURSt:PEAK?", "Flags"={"OPC Wait"=FALSE, "Dont check status"=FALSE, "*WAI"=FALSE}, "Check Status Callback"=""}, {"Level"=3, "Descriptive Name"="WLAN Fetch Crest Factor", "Class Only"=FALSE, "Data Type"=1, "Access"=0, "Identifier"="RSZVL_ATTR_WLAN_FETC_CRES", "Range Table"="", "Command"="FETC:BURS:CRES:{ModifMinMaxAver}?", "Read Callback"="", "Write Callback"="", "Range Callback"="", "Check Callback"="", "Rngtable Callback"="", "Coerce Callback"="", "User Callback"="", "Supported Models"="", "Instrument Options"="", "Repeated Capabilities"="", "Restricted 
